vi "温感调试助手.vi"() -> ()   [LabVIEW 2015]
uses:
  <vilib>/event_ctls.llb/eventvkey.ctl
  <vilib>/Instr/_visa.llb/VISA Find Search Mode.ctl
  <vilib>/Instr/_visa.llb/VISA Configure Serial Port (Instr).vi
panel:
  out "温度值":dbl
  out "队列输出":refnum<queue>
  in  "发送":bool
  in  "HEX发送":bool
  in  "发送区":string
  in  "获取温度":bool caption="ATE1"
  out "发送":string
  in  "窗口":string
  in  "清空显示":bool caption="清空"
  out "VISA":refnum<visa-resource-name>
  in  "端口":string(combo)="COM2"
  in  "波特率":string(combo)="115200"
  out "串口指示灯":bool caption="布尔"
  in  "串口开关":bool
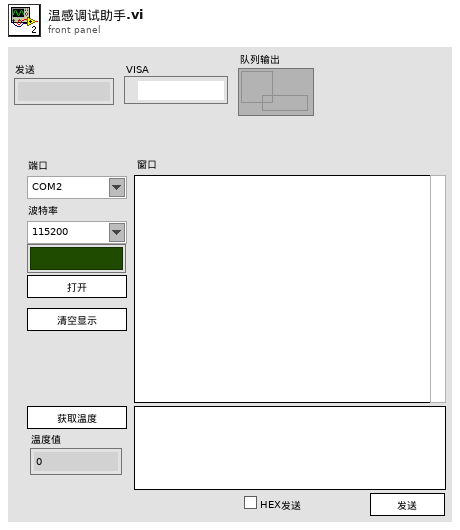
[diagram p1: front panel]
types:
  T1 = typedef "VISA Find Search Mode.ctl" = u32
  T2 = typedef "eventvkey.ctl" = enum16{"ASCII", "Enter", "Return", "Shift", "Ctrl", "Alt", "Cmd", "Opt", "Caps", "NumLock", "Clear", "Break", "Up", "Down", "Left", "Right", "Insert", "Delete", "Home", "End", "PageUp", "PageDown", "Escape", "Help", "Pause", "ScrollLock", "F1", "F2", "F3", "F4", "F5", "F6", "F7", "F8", "F9", "F10", "F11", "F12", "F13", "F14", "F15", "F16", "F17", "F18", "F19", "F20", "F21", "F22", "F23", "F24", "Play", "VolumeUp", "VolumeDown", "Mute", "Two Byte Char"}
  T3 = cluster{"Shift":bool, "Ctrl":bool, "Alt":bool, "Cmd":bool, "Opt":bool}
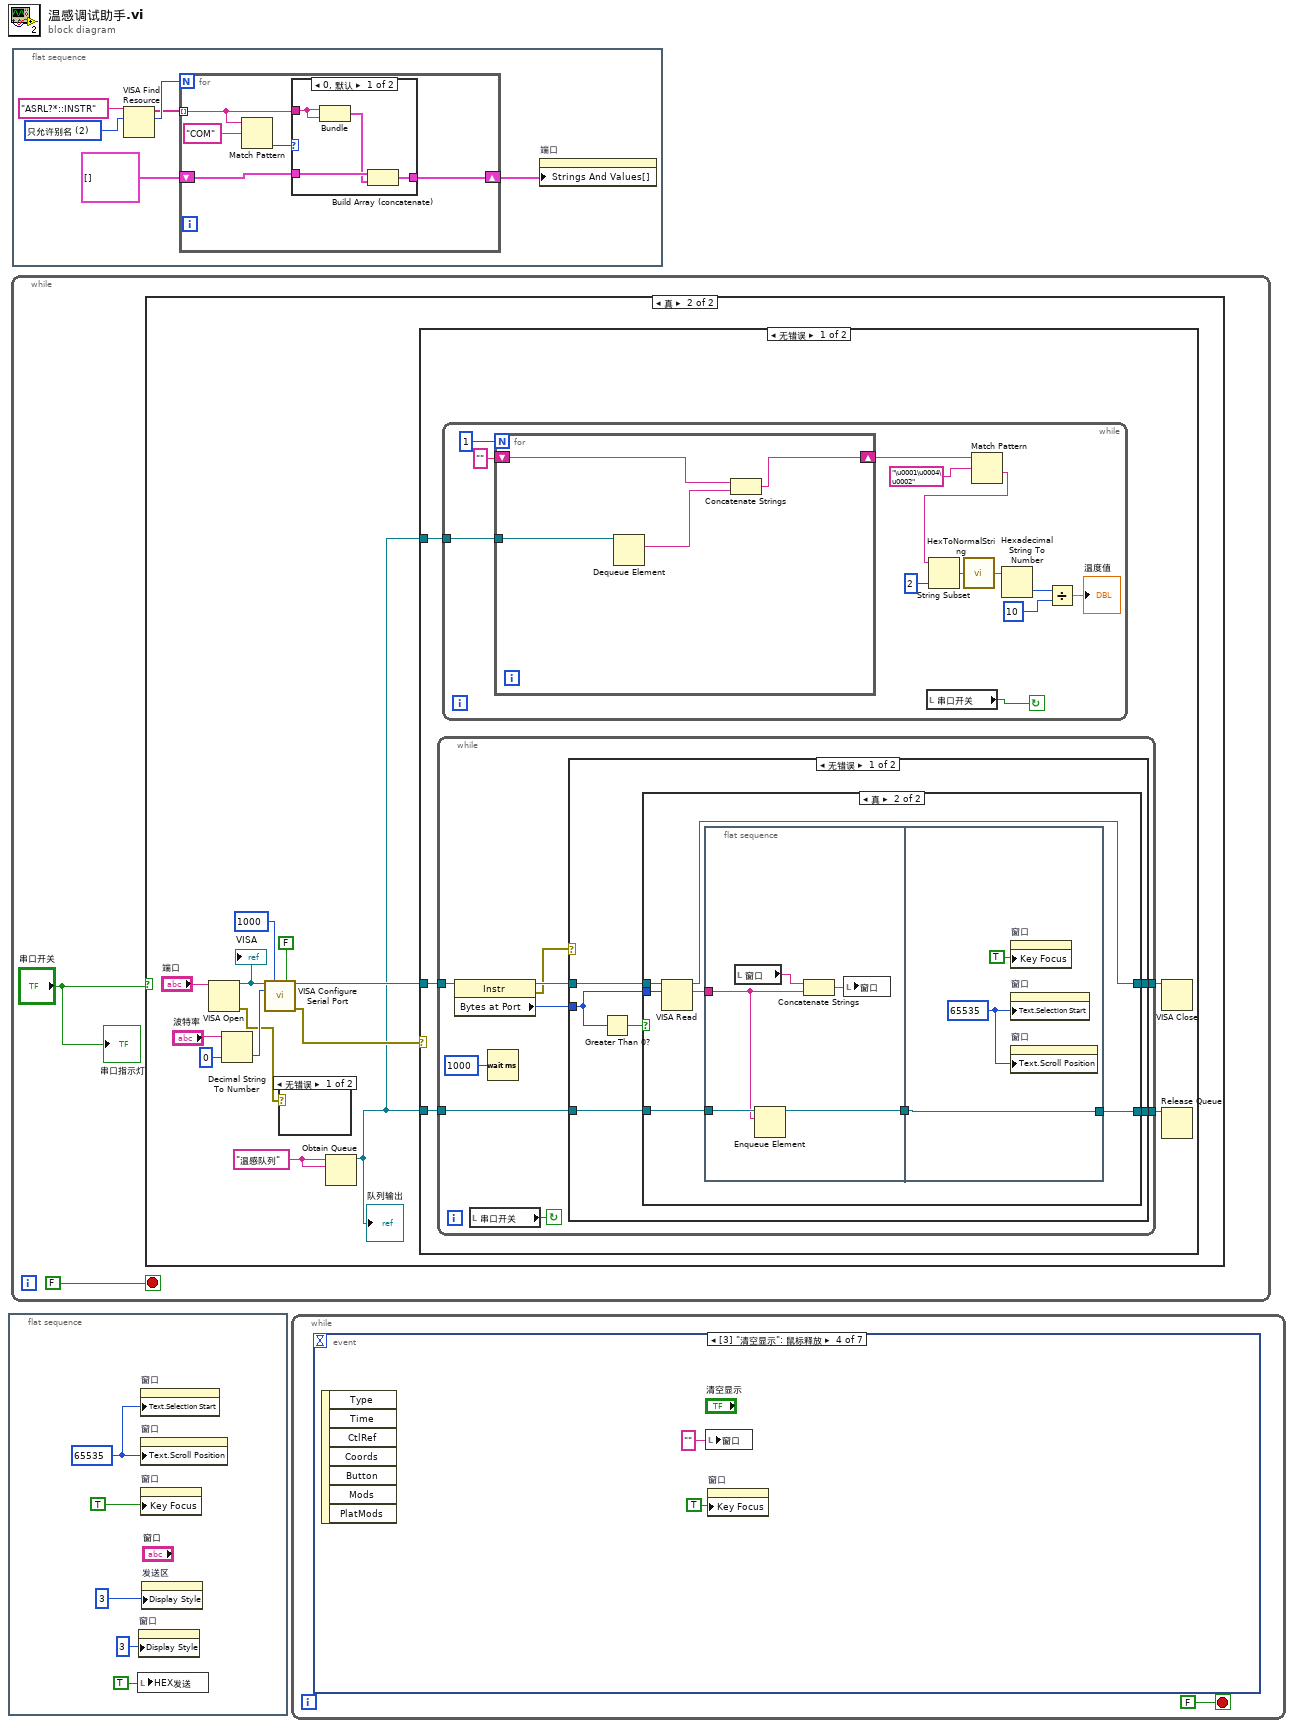
[diagram p0: block diagram]
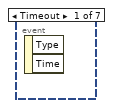
[diagram p3: hidden frame]
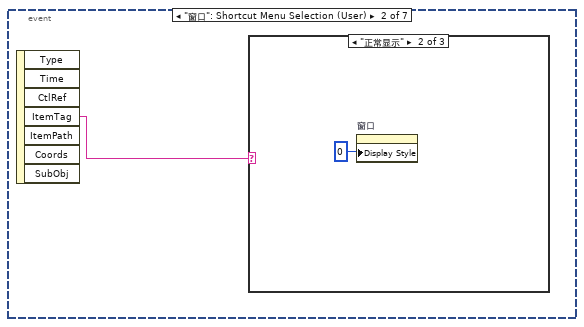
[diagram p4: hidden frame]
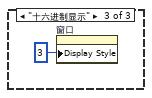
[diagram p6: hidden frame]
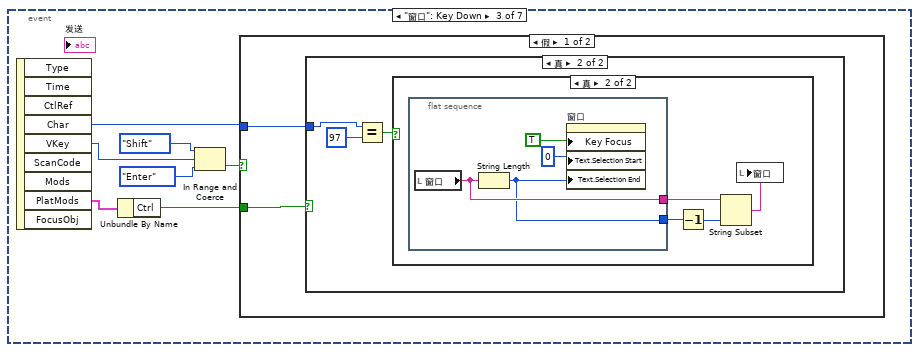
[diagram p7: hidden frame]
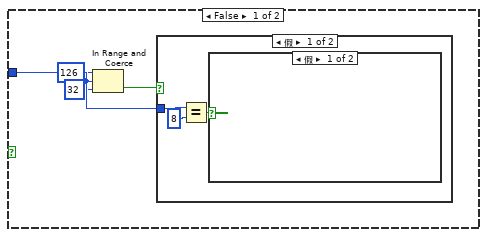
[diagram p8: hidden frame]
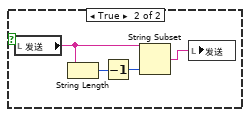
[diagram p9: hidden frame]
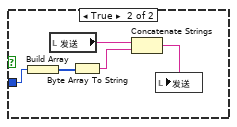
[diagram p10: hidden frame]
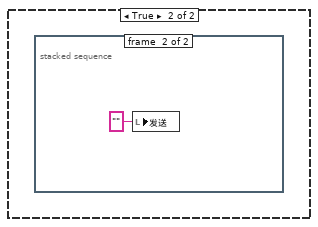
[diagram p12: hidden frame]
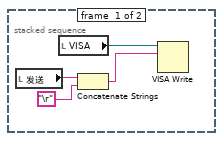
[diagram p13: hidden frame]
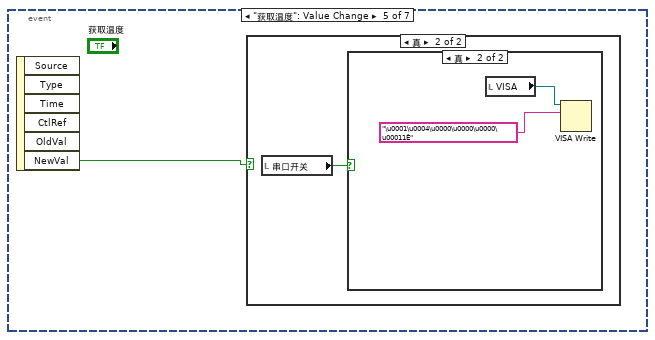
[diagram p14: hidden frame]
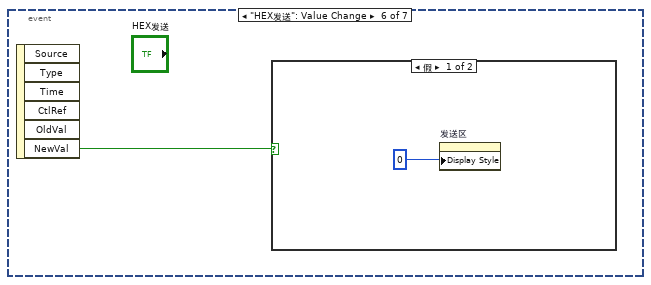
[diagram p17: hidden frame]
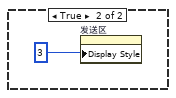
[diagram p18: hidden frame]
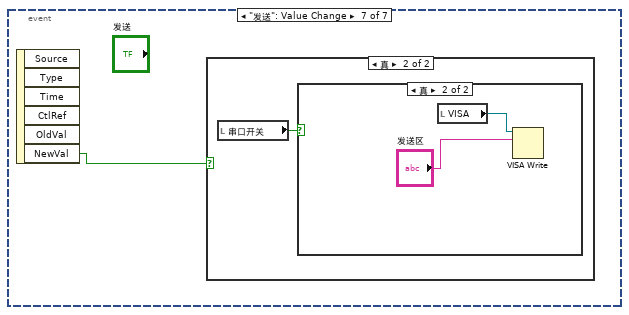
[diagram p19: hidden frame]
diagram:
  n1 = flat-sequence {
    frame #0 {
      w4 = u32 65535 ("文本.滚动条位置")
      n2 = local write "HEX发送"(TRUE) -> ()
      n3 = property on="窗口" class="Str"("Display Style"=u32 3 ("显示样式")) -> ()  [unwired: 2 in, 2 out]
      n4 = property on="窗口" class="Str"("Text.Selection Start"=w4) -> ()  [unwired: 2 in, 2 out]
      n5 = property on="窗口" class="Str"("Text.Scroll Position"=w4) -> ()  [unwired: 2 in, 2 out]
      n6 = property on="窗口" class="Str"("Key Focus"=TRUE ("键选中")) -> ()  [unwired: 2 in, 2 out]
      n7 = property on="发送区" class="Str"("Display Style"=3) -> ()  [unwired: 2 in, 2 out]
    }
  }
  n8 = while {
    stop <- FALSE stop-if-true
    n9 = case shown="真" "串口开关" {
      frame False {
        n10 = Wait (ms)(milliseconds to wait=u32 500 ("等待时间（毫秒）")) -> ()  [unwired: 1 out]
      }
      frame True {
        w10 = "温感队列"
        n11 = VISA Open(VISA resource name="端口") -> (VISA resource name=w20:refnum<visa-resource-name>, error out=w11:errorcluster)  [unwired: 4 in]
        "VISA" <- w20
        n12 = Decimal String To Number(string="波特率", default (0L)=u32 0 ("默认(0 I32)")) -> (number=w15:u32)  [unwired: 1 in, 1 out]
        n13 = call-poly "VISA Configure Serial Port"("VISA resource name"=w20, "timeout (10sec)"=u32 1000, "Enable Termination\nChar (T)"=FALSE ("Enable Termination\nChar (T)"), "baud rate (9600)"=w15) -> ("VISA resource name out"=w17:refnum<visa-resource-name>, "error out"=w12:errorcluster)  [unwired: 10 in]
        n14 = case shown="无错误" w11 {
          frame No Error {
          }
          frame Error {
          }
        }
        n15 = Obtain Queue(name (unnamed)=w10, element data type=w10) -> (queue out=w9:refnum<queue>)  [unwired: 3 in, 2 out]
        "队列输出" <- w9
        n16 = case shown="无错误" w12 {
          tunnel: w17 -> [w24 _]
          tunnel: w9 -> [w23 _]
          tunnel: w9 -> [w21 _]
          frame No Error {
            n17 = while {
              tunnel: [w49] -> w25
              tunnel: w24 -> [w47]
              tunnel: w23 -> [w44]
              tunnel: [w43] -> w22
              stop <- w51 continue-if-true
              n18 = property class="Instr"(reference=w47) -> (reference out=w50:refnum<visa-resource-name>, error out=w45:errorcluster, "Bytes at Port"=w46:u32)  [unwired: 1 in]
              n19 = local read "串口开关"() -> (w51:bool)
              n20 = Wait (ms)(milliseconds to wait=u32 1000 ("等待时间（毫秒）")) -> ()  [unwired: 1 out]
              n21 = case shown="无错误" w45 {
                tunnel: w50 -> [w57 w76]
                tunnel: [w56 w76] -> w49
                tunnel: w46 -> [w54 _]
                tunnel: w44 -> [w53 w75]
                tunnel: [w52 w75] -> w43
                frame No Error {
                  n22 = Greater Than 0?(x=w54) -> (x > 0?=w55:bool)
                  n23 = case shown="真" w55 {
                    tunnel: w57 -> [w59 w66]
                    tunnel: w54 -> [_ w65]
                    tunnel: [w59 w64] -> w56
                    tunnel: w53 -> [w58 w62]
                    tunnel: [w58 w60] -> w52
                    frame False {
                    }
                    frame True {
                      n24 = VISA Read(VISA resource name=w66, byte count=w65) -> (VISA resource name out=w64:refnum<visa-resource-name>, read buffer=w63:string)  [unwired: 1 in, 2 out]
                      n25 = flat-sequence {
                        tunnel: w63 -> [w68]
                        tunnel: w62 -> [w69]
                        tunnel: [w67] -> w61
                        tunnel: [w72] -> w60
                        tunnel: w61 -> [w72]
                        frame #0 {
                          n26 = local read "窗口"() -> (w70:string)
                          n27 = Enqueue Element(queue=w69, element=w68) -> (queue out=w67:refnum<queue>)  [unwired: 2 in, 2 out]
                          n28 = Concatenate Strings(w70, w68) -> (w71:string)
                          n29 = local write "窗口"(w71) -> ()
                        }
                        frame #1 {
                          w73 = u32 65535 ("文本.选择区域:起始")
                          n30 = property on="窗口" class="Str"("Key Focus"=TRUE ("键选中")) -> ()  [unwired: 2 in, 2 out]
                          n31 = property on="窗口" class="Str"("Text.Selection Start"=w73) -> ()  [unwired: 2 in, 2 out]
                          n32 = property on="窗口" class="Str"("Text.Scroll Position"=w73) -> ()  [unwired: 2 in, 2 out]
                        }
                      }
                    }
                  }
                }
                frame Error {
                }
              }
            }
            n33 = while {
              tunnel: w21 -> [w27]
              stop <- w28 continue-if-true
              n34 = for {
                N: 1 -> [_]
                shift-right: [w40] -> w37
                shift-left: "" -> [w41]
                tunnel: w27 -> [w39]
                n35 = Dequeue Element(queue=w39) -> (element=w42:string)  [unwired: 2 in, 3 out]
                n36 = Concatenate Strings(w41, w42) -> (w40:string)
              }
              n37 = local read "串口开关"() -> (w28:bool)
              n38 = Match Pattern(string=w37, regular expression="\u0001\u0004\u0002") -> (after substring=w35:string)  [unwired: 1 in, 3 out]
              n39 = String Subset(string=w35, length (rest)=2) -> (substring=w33:string)  [unwired: 1 in]
              n40 = call "HexToNormalString.vi"("Hex Display"=w33) -> ("Normal Display"=w32:string)  [unwired: 14 in]
              n41 = Hexadecimal String To Number(string=w32) -> (number=w31:u32)  [unwired: 2 in, 1 out]
              n42 = Divide(x=w31, y=10) -> (x/y=→"温度值":dbl)
            }
            n43 = VISA Close(VISA resource name=w25) -> ()  [unwired: 1 in, 1 out]
            n44 = Release Queue(queue=w22) -> ()  [unwired: 2 in, 3 out]
          }
          frame Error {
            n45 = flat-sequence {
              frame #0 {
                n46 = local read "端口"() -> (w79:string)
                n47 = Concatenate Strings(w79, "打开失败！" ("字符串")) -> (w77:string)
                n48 = One Button Dialog(message=w77) -> ()  [unwired: 1 in, 1 out]
              }
              frame #1 {
                n49 = local write "串口开关"(FALSE ("串口开关")) -> ()
              }
            }
          }
        }
      }
    }
    "串口指示灯" <- "串口开关"
  }
  n50 = flat-sequence {
    frame #0 {
      w83 = T1 2 items=["仅允许规范名称"=0, "只允许别名"=2, "包含匹配别名"=3, "包含所有别名"=4] ("Search Mode")
      n51 = VISA Find Resource(10:w83, 11:"ASRL?*::INSTR") -> (2:w85:u32, 3:w84:string[])  [unwired: 1 in, 1 out]
      n52 = for {
        N: w85 -> [_]
        tunnel: w84 -> [w89] mode=indexing
        shift-right: [w88] -> w81
        shift-left: cluster{string, string}[] [] -> [w87]
        n53 = Match Pattern(string=w89, regular expression="COM" ("正则表达式")) -> (offset past match=w90:i32)  [unwired: 1 in, 3 out]
        n54 = case shown="0, 默认" w90 {
          tunnel: w87 -> [w95 w96]
          tunnel: w89 -> [w93 _]
          tunnel: [w94 w96] -> w88
          frame 0, Default {
            n55 = Bundle(w93, w93) -> (w92:cluster{string, string})  [unwired: 1 in]
            n56 = Build Array (concatenate)(w95, w92) -> (w94:cluster{string, string}[])
          }
          frame -1 {
          }
        }
      }
      n57 = property on="端口" class="CmbBox"("Strings And Values[]"=w81) -> ()  [unwired: 2 in, 2 out]
    }
  }
  n58 = while {
    stop <- FALSE stop-if-true
    n59 = event shown="[3] \"清空显示\": 鼠标释放" {
      selector: _ -> [_ _ _ _ _ _ _]
      dyn-events: _ -> [_ _ _ _ _ _ _]
      timeout: _ -> [_ _ _ _ _ _ _]
      event Timeout {
        n60 = event-data() -> ()  [unwired: 1 in, 2 out]
      }
      event "窗口": Shortcut Menu Selection (User) {
        n61 = event-data() -> ("ItemTag"=w98:string)  [unwired: 1 in, 6 out]
        n62 = case shown="\"正常显示\"" w98 {
          frame "假", Default {
          }
          frame "正常显示" {
            n63 = property on="窗口" class="Str"("Display Style"=u32 0 ("显示样式")) -> ()  [unwired: 2 in, 2 out]
          }
          frame "十六进制显示" {
            n64 = property on="窗口" class="Str"("Display Style"=u32 3 ("显示样式")) -> ()  [unwired: 2 in, 2 out]
          }
        }
      }
      event "窗口": Key Down {
        n65 = event-data() -> ("Char"=w107:i16, "VKey"=w103:T2, "PlatMods"=w102:T3)  [unwired: 1 in, 6 out]
        n66 = Unbundle By Name(w102) -> ("Ctrl"=w101:bool)
        n67 = In Range and Coerce(upper limit=eventvkey."Shift" ("上限"), x=w103, lower limit=eventvkey."Enter" ("下限")) -> (In Range?=w104:bool)  [unwired: 1 out]
        n68 = case shown="假" w104 {
          tunnel: w107 -> [w109 _]
          tunnel: w101 -> [w108 _]
          frame False {
            n69 = case shown="真" w108 {
              tunnel: w109 -> [w113 w128]
              frame False {
                n70 = In Range and Coerce(upper limit=i16 126 ("上限"), x=w113, lower limit=i16 32 ("下限")) -> (In Range?=w112:bool)  [unwired: 1 out]
                n71 = case shown="假" w112 {
                  tunnel: w113 -> [w116 w122]
                  frame False {
                    n72 = Equal?(x=w116, y=i16 8) -> (x = y?=w114:bool)
                    n73 = case shown="假" w114 {
                      frame False {
                      }
                      frame True {
                        n74 = local read "发送"() -> (w118:string)
                        n75 = String Length(string=w118) -> (length=w119:i32)
                        n76 = Decrement(x=w119) -> (x-1=w120:i32)
                        n77 = String Subset(string=w118, length (rest)=w120) -> (substring=w117:string)  [unwired: 1 in]
                        n78 = local write "发送"(w117) -> ()
                      }
                    }
                  }
                  frame True {
                    n79 = Build Array(w122) -> (w123:i16[])
                    n80 = local read "发送"() -> (w125:string)
                    n81 = Byte Array To String(unsigned byte array=w123) -> (string=w121:string)
                    n82 = Concatenate Strings(w125, w121) -> (w124:string)
                    n83 = local write "发送"(w124) -> ()
                  }
                }
              }
              frame True {
                n84 = Equal?(x=w128, y=i16 97) -> (x = y?=w126:bool)
                n85 = case shown="真" w126 {
                  frame False {
                  }
                  frame True {
                    n86 = flat-sequence {
                      tunnel: [w134] -> w132
                      tunnel: [w133] -> w130
                      frame #0 {
                        n87 = local read "窗口"() -> (w134:string)
                        n88 = String Length(string=w134) -> (length=w133:i32)
                        n89 = property on="窗口" class="Str"("Key Focus"=TRUE ("键选中"), "Text.Selection Start"=u32 0 ("文本.选择区域:起始"), "Text.Selection End"=w133) -> ()  [unwired: 2 in, 2 out]
                      }
                    }
                    n90 = Decrement(x=w130) -> (x-1=w131:i32)
                    n91 = String Subset(string=w132, length (rest)=w131) -> (substring=w129:string)  [unwired: 1 in]
                    n92 = local write "窗口"(w129) -> ()
                  }
                }
              }
            }
          }
          frame True {
            n93 = stacked-sequence {
              frame #0 {
                n94 = local read "发送"() -> (w138:string)
                n95 = local read "VISA"() -> (w140:refnum<visa-resource-name>)
                n96 = Concatenate Strings(w138, "\r") -> (w139:string)
                n97 = VISA Write(VISA resource name=w140, write buffer=w139) -> ()  [unwired: 1 in, 3 out]
              }
              frame #1 {
                n98 = local write "发送"("" ("发送")) -> ()
              }
            }
          }
        }
      }
      event "清空显示": Mouse Up {
        n99 = event-data() -> ()  [unwired: 1 in, 7 out]
        n100 = local write "窗口"("") -> ()
        n101 = property on="窗口" class="Str"("Key Focus"=TRUE ("键选中")) -> ()  [unwired: 2 in, 2 out]
      }
      event "获取温度": Value Change {
        n102 = event-data() -> ("NewVal"=w144:bool)  [unwired: 1 in, 5 out]
        n103 = case shown="真" w144 {
          frame False {
          }
          frame True {
            n104 = local read "串口开关"() -> (w145:bool)
            n105 = case shown="真" w145 {
              frame False {
              }
              frame True {
                n106 = local read "VISA"() -> (w147:refnum<visa-resource-name>)
                n107 = VISA Write(VISA resource name=w147, write buffer="\u0001\u0004\u0000\u0000\u0000\u00011Ê") -> ()  [unwired: 1 in, 3 out]
              }
            }
          }
        }
      }
      event "HEX发送": Value Change {
        n108 = event-data() -> ("NewVal"=w148:bool)  [unwired: 1 in, 5 out]
        n109 = case shown="假" w148 {
          frame False {
            n110 = property on="发送区" class="Str"("Display Style"=0) -> ()  [unwired: 2 in, 2 out]
          }
          frame True {
            n111 = property on="发送区" class="Str"("Display Style"=3) -> ()  [unwired: 2 in, 2 out]
          }
        }
      }
      event "发送": Value Change {
        n112 = event-data() -> ("NewVal"=w151:bool)  [unwired: 1 in, 5 out]
        n113 = case shown="真" w151 {
          frame False {
          }
          frame True {
            n114 = local read "串口开关"() -> (w152:bool)
            n115 = case shown="真" w152 {
              frame False {
              }
              frame True {
                n116 = local read "VISA"() -> (w154:refnum<visa-resource-name>)
                n117 = VISA Write(VISA resource name=w154, write buffer="发送区") -> ()  [unwired: 1 in, 3 out]
              }
            }
          }
        }
      }
    }
  }
